vi "Error Message.vi"(0 "VISA resource name":refnum<visa-resource-name>, 5 "Type of Dialog (1: OK Msg)":T1(ring)=enum."OK Message", 7 "User-Defined Codes":i32[](array[numeric]), 9 "User-Defined Descriptions":string[](array[string]), 11 "error in (no error)":errorcluster {"code" format="%.0x"}) -> (3 "Status":bool, 4 "VISA resource name out":refnum<visa-resource-name>, 8 "Error Code (0)":i32, 10 "Error Message (empty)":string, 15 "error out":errorcluster {"code" format="%.0x"})   [LabVIEW 2014, in "Eurotherm 35xx Series.lvlib"]
doc: "This VI contains all the instrument specific error codes and descriptions. Use this VI after executing several instrument driver VIs to recognize and display any errors that may have occurred."
uses:
  <instrlib>/Eurotherm 35xx Series/Eurotherm 35xx Series.lvlib
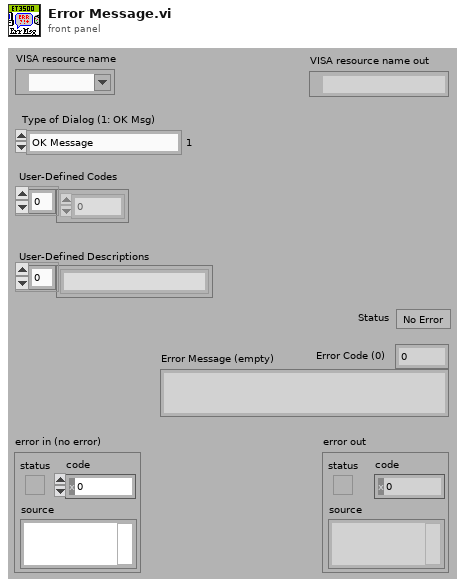
[diagram p1: front panel]
types:
  T1 = enum16{"No Dialog", "OK Message", "Continue or Stop Message"}
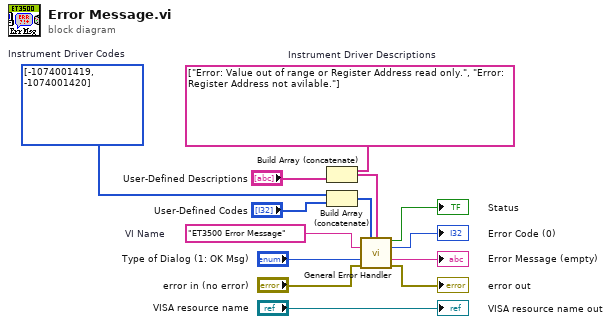
[diagram p0: block diagram]
diagram:
  w6 = i32[] [-1074001419, -1074001420]  # Instrument Driver Codes
  w7 = string[] ["Error: Value out of range or Register Address read only.", "Error: Register Address not avilable."]  # Instrument Driver Descriptions
  w11 = "ET3500 Error Message"  # VI Name
  n1 = Build Array (concatenate)(w7, "User-Defined Descriptions") -> (w5:string[])
  n2 = Build Array (concatenate)(w6, "User-Defined Codes") -> (w4:i32[])
  n3 = call <vilib>:"General Error Handler.vi"("[user-defined codes]"=w4, "[user-defined descriptions]"=w5, "[error source] (\" \")"=w11, "type of dialog (OK msg:1)"="Type of Dialog (1: OK Msg)", "error in (no error)"="error in (no error)") -> ("error?"=→"Status":bool, "code out"=→"Error Code (0)":i32, "message"=→"Error Message (empty)":string, "error out"=→"error out":errorcluster)  [unwired: 6 in, 1 out]
  "VISA resource name out" <- "VISA resource name"
